vi "Start Sync.vi"(8 "error in (no error)":errorcluster, 10 "current time":timestamp, 11 "gRPC Server in":refnum<class "OCV3.lvclass">) -> (0 "error out":errorcluster, 3 "gRPC Server out":refnum<class "OCV3.lvclass">)   [LabVIEW 2019, in "OCV3.lvlib" / "OCV3.lvclass"]
uses:
  OCV3.lvclass
  OCV3.lvclass/OCV3.ctl
  RPC Messages/measurementservice_OCVRaw/measurementservice_OCVRaw_Data.ctl
  RPC Messages/measurementservice_ErrorOut/measurementservice_ErrorOut_Data.ctl
  RPC Messages/measurementservice_OCVData/measurementservice_OCVData_Data.ctl
  RPC Messages/measurementservice_QueryResponse/measurementservice_QueryResponse_Data.ctl
  RPC Messages/measurementservice_ACIRData/measurementservice_ACIRData_Data.ctl
  RPC Messages/measurementservice_ACIRRaw/measurementservice_ACIRRaw_Data.ctl
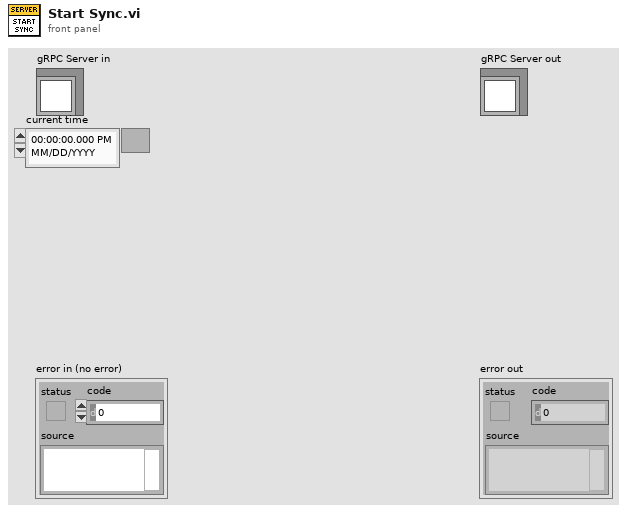
[diagram p1: front panel]
types:
  T1 = typedef "OCV3.lvlib/OCV3.lvclass/measurementservice_ErrorOut_Data.ctl" = cluster{"errCode":i32, "errMessage":string}
  T2 = typedef "OCV3.lvlib/OCV3.lvclass/measurementservice_OCVData_Data.ctl" = cluster{"data":T3[]}
  T3 = typedef "OCV3.lvlib/OCV3.lvclass/measurementservice_OCVRaw_Data.ctl" = cluster{"battery1voltage":sgl, "battery2voltage":sgl, "battery3voltage":sgl, "battery4voltage":sgl, "battery5voltage":sgl, "battery6voltage":sgl, "battery7voltage":sgl, "battery8voltage":sgl, "battery9voltage":sgl, "battery10voltage":sgl, "battery11voltage":sgl, "battery12voltage":sgl, "battery13voltage":sgl, "battery14voltage":sgl, "battery15voltage":sgl, "battery16voltage":sgl, "battery17voltage":sgl, "battery18voltage":sgl, "battery19voltage":sgl, "battery20voltage":sgl, "battery21voltage":sgl, "battery22voltage":sgl, "battery23voltage":sgl, "battery24voltage":sgl, "error":T1}
  T4 = typedef "OCV3.lvlib/OCV3.lvclass/measurementservice_QueryResponse_Data.ctl" = cluster{"message":string, "status":i32}
  T5 = typedef "OCV3.lvlib/OCV3.lvclass/measurementservice_ACIRRaw_Data.ctl" = cluster{"Impedance":sgl, "Real":sgl, "Imaginery":sgl, "error":T1}
  T6 = typedef "OCV3.lvlib/OCV3.lvclass/measurementservice_ACIRData_Data.ctl" = cluster{"data":T5[]}
  T7 = typedef "OCV3.lvlib/OCV3.lvclass/Server gRPC UEs.ctl" = cluster{"Invoke gRPC UE":refnum<user-event>, "Query gRPC UE":refnum<user-event>, "PerformOCVMeasurement gRPC UE":refnum<user-event>, "PerformACIRMeasurement gRPC UE":refnum<user-event>, "StreamOCVMeasurement gRPC UE":refnum<user-event>, "Register gRPC UE":refnum<user-event>}
  T8 = typedef "OCV3.lvlib/gprc-lvsupport.lvlib/grpcId.ctl" = u64
  T9 = typedef "OCV3.lvlib/OCV3.lvclass/measurementservice_QueryRequest_Data.ctl" = cluster{"query":string}
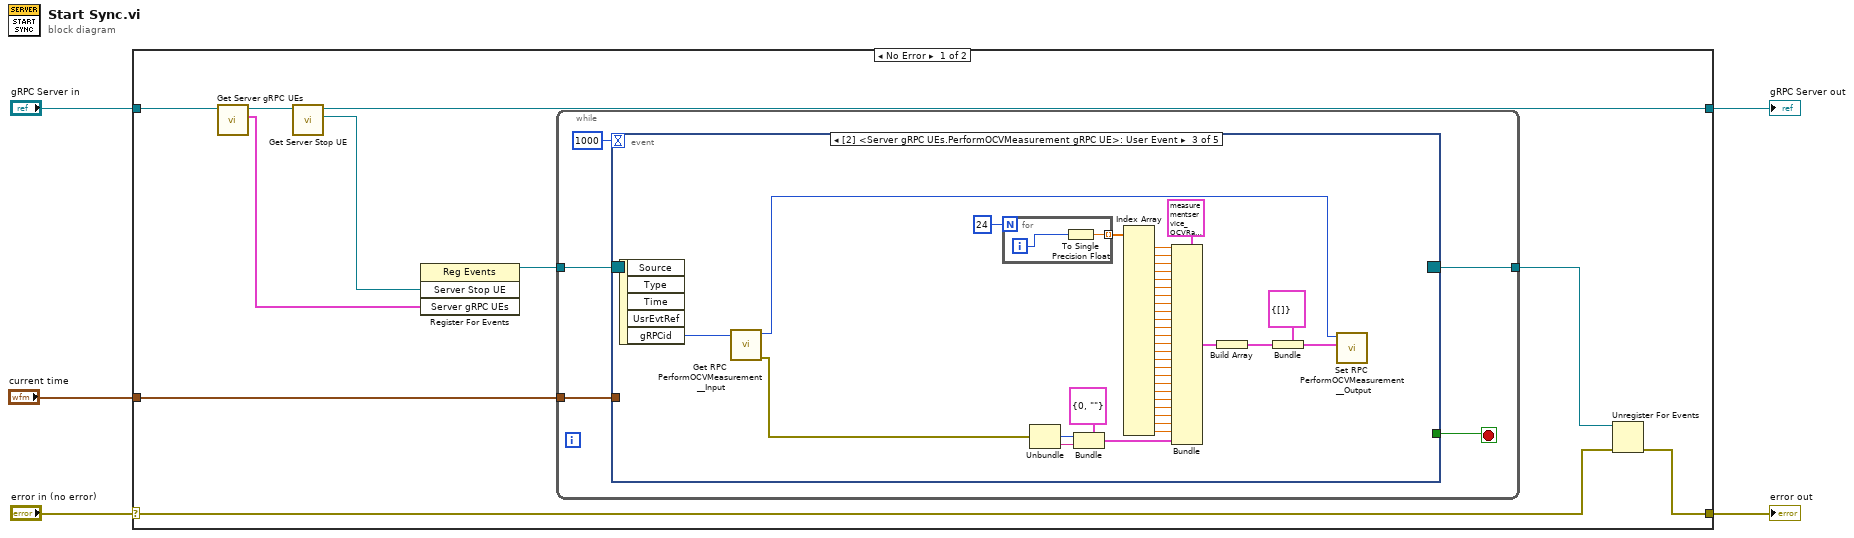
[diagram p0: block diagram]
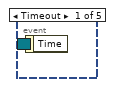
[diagram p2: hidden frame]
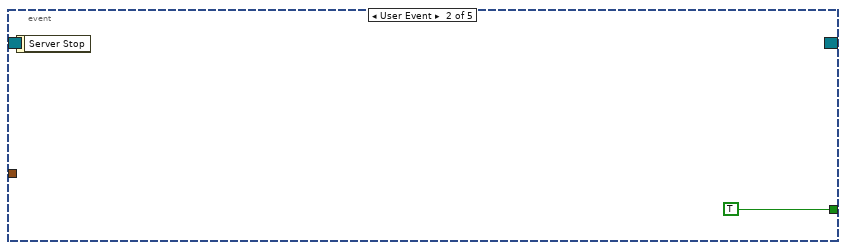
[diagram p3: hidden frame]
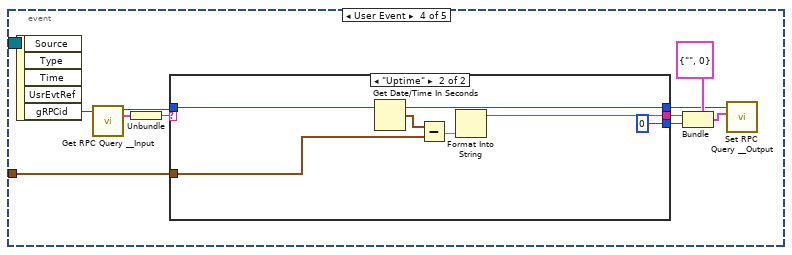
[diagram p4: hidden frame]
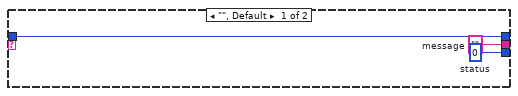
[diagram p5: hidden frame]
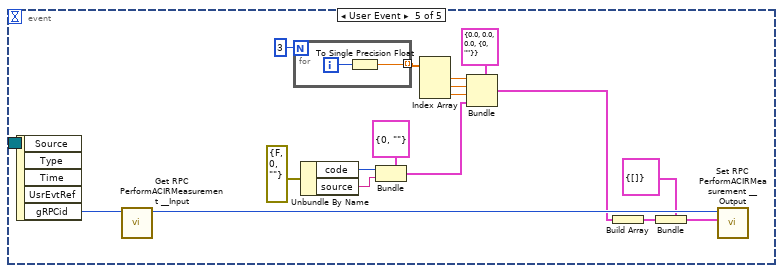
[diagram p6: hidden frame]
diagram:
  n1 = case shown="No Error" "error in (no error)" {
    selector: "error in (no error)" -> [w8 w101]
    tunnel: [w7 w101] -> w4
    tunnel: [w11 w100] -> w2
    tunnel: "gRPC Server in" -> [w15 w100]
    tunnel: "current time" -> [w6 _]
    frame No Error {
      n2 = call "Get Server gRPC UEs.vi"("OOP Server in"=w15) -> ("Server gRPC UEs"=w12:T7, "OOP Server out"=w14:refnum<class "OCV3.lvclass">)  [unwired: 9 in]
      n3 = call "Get Server Stop UE.vi"("OOP Server in"=w14) -> ("Server Stop UE"=w13:refnum<user-event>, "OOP Server out"=w11:refnum<class "OCV3.lvclass">)  [unwired: 9 in]
      n4 = register-events(w13, w12) -> (reference out=w10:refnum<event-registration>)  [unwired: 2 in, 1 out]
      n5 = while {
        tunnel: w10 -> [w20]
        tunnel: [w18] -> w9
        tunnel: w6 -> [w16]
        stop <- w19 stop-if-true
        n6 = event "RPC Methods Event Structure" shown="[2] <Server gRPC UEs.PerformOCVMeasurement gRPC UE>: User Event" {
          selector: w20 -> [_ _ _ _ _]
          dyn-events: [_ _ _ _ _] -> w18
          timeout: 1000 -> [_ _ _ _ _]
          tunnel: [_ TRUE _ _ _] -> w19
          tunnel: w16 -> [_ _ _ w62 _]
          event Timeout {
            n7 = event-data() -> ()  [unwired: 1 in, 1 out]
          }
          event User Event {
            n8 = event-data() -> ()  [unwired: 1 in, 1 out]
          }
          event User Event {
            n9 = event-data() -> ("gRPCid"=w23:T8)  [unwired: 1 in, 4 out]
            n10 = call "Get RPC PerformOCVMeasurement __Input.vi"("gRPCid in"=w23) -> ("error out"=w22:errorcluster, "gRPCid out"=w59:T8)  [unwired: 8 in, 1 out]
            n11 = for {
              N: 24 -> [_]
              tunnel: [w61] -> w52 mode=indexing
              i -> [w60]
              n12 = To Single Precision Float(number=w60) -> (single precision float=w61:sgl)
            }
            n13 = Unbundle(w22) -> ("code"=w26:i32, "source"=w25:string)  [unwired: 1 out]
            n14 = Bundle(cluster=T1 {"errCode"=0, "errMessage"=""} ("measurementservice_ErrorOut_Data"), "errCode"=w26, "errMessage"=w25) -> (w24:T1)
            n15 = Index Array(array=w52) -> (element #1=w51:sgl, element #2=w50:sgl, element #3=w49:sgl, element #4=w48:sgl, element #5=w47:sgl, element #6=w46:sgl, element #7=w45:sgl, element #8=w44:sgl, element #9=w43:sgl, element #10=w42:sgl, element #11=w41:sgl, element #12=w40:sgl, element #13=w39:sgl, element #14=w38:sgl, element #15=w37:sgl, element #16=w36:sgl, element #17=w35:sgl, element #18=w34:sgl, element #19=w33:sgl, element #20=w32:sgl, element #21=w31:sgl, element #22=w30:sgl, element #23=w29:sgl, element #24=w28:sgl)  [unwired: 24 in]
            n16 = Bundle(cluster=T3 {"battery1voltage"=0.0, "battery2voltage"=0.0, "battery3voltage"=0.0, "battery4voltage"=0.0, "battery5voltage"=0.0, "battery6voltage"=0.0, "battery7voltage"=0.0, "battery8voltage"=0.0, "battery9voltage"=0.0, "battery10voltage"=0.0, "battery11voltage"=0.0, "battery12voltage"=0.0, "battery13voltage"=0.0, "battery14voltage"=0.0, "battery15voltage"=0.0, "battery16voltage"=0.0, "battery17voltage"=0.0, "battery18voltage"=0.0, "battery19voltage"=0.0, "battery20voltage"=0.0, "battery21voltage"=0.0, "battery22voltage"=0.0, "battery23voltage"=0.0, "battery24voltage"=0.0, "error"={"errCode"=0, "errMessage"=""}} ("measurementservice_OCVRaw_Data"), "battery1voltage"=w51, "battery2voltage"=w50, "battery3voltage"=w49, "battery4voltage"=w48, "battery5voltage"=w47, "battery6voltage"=w46, "battery7voltage"=w45, "battery8voltage"=w44, "battery9voltage"=w43, "battery10voltage"=w42, "battery11voltage"=w41, "battery12voltage"=w40, "battery13voltage"=w39, "battery14voltage"=w38, "battery15voltage"=w37, "battery16voltage"=w36, "battery17voltage"=w35, "battery18voltage"=w34, "battery19voltage"=w33, "battery20voltage"=w32, "battery21voltage"=w31, "battery22voltage"=w30, "battery23voltage"=w29, "battery24voltage"=w28, "error"=w24) -> (w57:T3)
            n17 = Build Array(w57) -> (w55:T3[])
            n18 = Bundle(cluster=T2 {"data"=[]} ("Message Data"), "data"=w55) -> (w54:T2)
            n19 = call "Set RPC PerformOCVMeasurement __Output.vi"("Message Data"=w54, "gRPCid in"=w59) -> ()  [unwired: 9 in, 1 out]
          }
          event User Event {
            n20 = event-data() -> ("gRPCid"=w63:T8)  [unwired: 1 in, 4 out]
            n21 = call "Get RPC Query __Input.vi"("gRPCid in"=w63) -> ("Message Data"=w70:T9, "gRPCid out"=w71:T8)  [unwired: 8 in, 1 out]
            n22 = Unbundle(w70) -> ("query"=w69:string)
            n23 = case shown="\"Uptime\"" w69 {
              tunnel: w71 -> [w74 w77]
              tunnel: [w74 w77] -> w64
              tunnel: [w73 w78] -> w66
              tunnel: [w72 0 ("status")] -> w65
              tunnel: w62 -> [_ w75]
              frame "", Default {
                w72 = 0  # status
                w73 = ""  # message
              }
              frame "Uptime" {
                n24 = Get Date/Time In Seconds() -> (seconds since 1Jan1904=w80:timestamp)
                n25 = Subtract(x=w80, y=w75) -> (x-y=w79:dbl)
                n26 = Format Into String(w79) -> (resulting string=w78:string)  [unwired: 3 in, 1 out]
              }
            }
            n27 = Bundle(cluster=T4 {"message"="", "status"=0} ("Message Data"), "message"=w66, "status"=w65) -> (w67:T4)
            n28 = call "Set RPC Query __Output.vi"("Message Data"=w67, "gRPCid in"=w64) -> ()  [unwired: 9 in, 1 out]
          }
          event User Event {
            n29 = event-data() -> ("gRPCid"=w81:T8)  [unwired: 1 in, 4 out]
            n30 = call "Get RPC PerformACIRMeasurement __Input.vi"("gRPCid in"=w81) -> ("gRPCid out"=w95:T8)  [unwired: 8 in, 2 out]
            n31 = for {
              N: 3 -> [_]
              tunnel: [w99] -> w85 mode=indexing
              i -> [w98]
              n32 = To Single Precision Float(number=w98) -> (single precision float=w99:sgl)
            }
            n33 = Unbundle By Name(errorcluster {"status"=FALSE, "code"=0, "source"=""} ("error in (no error)")) -> ("code"=w88:i32, "source"=w87:string)
            n34 = Bundle(cluster=T1 {"errCode"=0, "errMessage"=""} ("measurementservice_ErrorOut_Data"), "errCode"=w88, "errMessage"=w87) -> (w86:T1)
            n35 = Index Array(array=w85) -> (element #1=w84:sgl, element #2=w83:sgl, element #3=w82:sgl)  [unwired: 3 in]
            n36 = Bundle(cluster=T5 {"Impedance"=0.0, "Real"=0.0, "Imaginery"=0.0, "error"={"errCode"=0, "errMessage"=""}} ("measurementservice_ACIRRaw_Data"), "Impedance"=w84, "Real"=w83, "Imaginery"=w82, "error"=w86) -> (w90:T5)
            n37 = Build Array(w90) -> (w91:T5[])
            n38 = Bundle(cluster=T6 {"data"=[]} ("Message Data"), "data"=w91) -> (w93:T6)
            n39 = call "Set RPC PerformACIRMeasurement __Output.vi"("Message Data"=w93, "gRPCid in"=w95) -> ()  [unwired: 9 in, 1 out]
          }
        }
      }
      n40 = Unregister For Events(event registration refnum=w9, error in=w8) -> (error out=w7:errorcluster)
    }
    frame Error {
    }
  }
  "error out" <- w4
  "gRPC Server out" <- w2
